vi "Begin.vi"() -> (0 "error out":errorcluster)   [LabVIEW 2013]
doc: "Called before other user functions, this VI is expected to open initial I/O refnums, load in file data, and do all program initialization. Notice that the <B>error out</B> terminal is simply used for data flow. Wiring it to other structures or subVIs ensures that this VI runs first."
uses:
  <vilib>/Rock Robotics/WPI/DriverStation/WPI_DriverStationRobotMode2.ctl
  Robot Global Data.vi
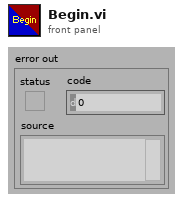
[diagram p1: front panel]
types:
  T1 = typedef "WPI_DriverStationRobotMode2.ctl" = enum16{"Autonomous Disabled", "Autonomous Enabled", "Teleop Disabled", "Teleop Enabled", "Timeout", "Finish", "Test Disabled", "Test Enabled"}
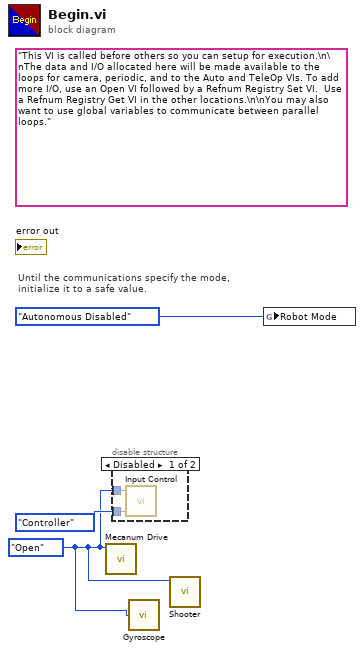
[diagram p0: block diagram]
diagram:
  w1 = enum16{"Open", "Run", "End"}."Open" ("State Control")
  (unwired) "This VI is called before others so you can setup for execution.\n\nThe data and I/O allocated here will be made available to the loops for camera, periodic, and to the Auto and TeleOp VIs. To add more I/O, use an Open VI followed by a Refnum Registry Set VI.  Use a Refnum Registry Get VI in the other locations.\n\nYou may also want to use global variables to communicate between parallel loops."
  # "Until the communications specify the mode,\ninitialize it to a safe value."
  n1 = call "Mecanum Drive.vi"("State Control"=w1) -> ()  [unwired: 3 in]
  n2 = disable-structure shown="Disabled" {
    disable-tunnel: enum16{"Joysticks", "Controller"}."Controller" ("Device") -> [w5 _]
    disable-tunnel: w1 -> [w4 _]
    frame Disabled {
      n3 = call "Input Control.vi"("Device"=w5, "State"=w4) -> ()  [unwired: 1 in, 3 out]
    }
    frame Enabled {
    }
  }
  n4 = call "Gyroscope.vi"("State Control"=w1) -> ()  [unwired: 1 in]
  n5 = call "Shooter.vi"("State Control"=w1) -> ()  [unwired: 11 in]
  n6 = global write "Robot Global Data.vi" "Robot Mode"(WPI_DriverStationRobotMode2."Autonomous Disabled" ("Robot Mode")) -> ()
